vi "LHF.DB.Mongo.Collection.JSON.Aggregate.vi"(6 "Extract _id (T)":bool=TRUE, 8 "error in (no error)":errorcluster, 9 "Operations":variant[](array[variant]), 10 "Collection":string, 11 "LHF.DB.Mongo in":refnum<class "LHF.DB.Mongo.lvclass">) -> (0 "error out":errorcluster, 1 "_id Array":string[](array[string]), 2 "Documents":string[](array[string]), 3 "LHF.DB.Mongo out":refnum<class "LHF.DB.Mongo.lvclass">)   [LabVIEW 2013, in "LHF.DB.Mongo.lvclass"]
doc: "return type: wire cluster of expected document output, then variant to data with documents output. use cluster element's name to choose what document field you're expecting\noperations: wire array of cluster variant, name the cluster variant with the desired aggregation operation as $project or $match then use element names to setup pipeline."
uses:
  LHF.DB.Mongo.lvclass
  C:/Users/Ricardo/Desktop/Projetos/LabVIEW-MongoDB/src/Driver/MongoDB.Bson.dll
  Driver/MongoDB.Bson.dll
  <userlib>/_OpenG.lib/string/string.llb/Trim Whitespace (String)__ogtk.vi
  <vilib>/Utility/VariantDataType/VariantType.lvlib
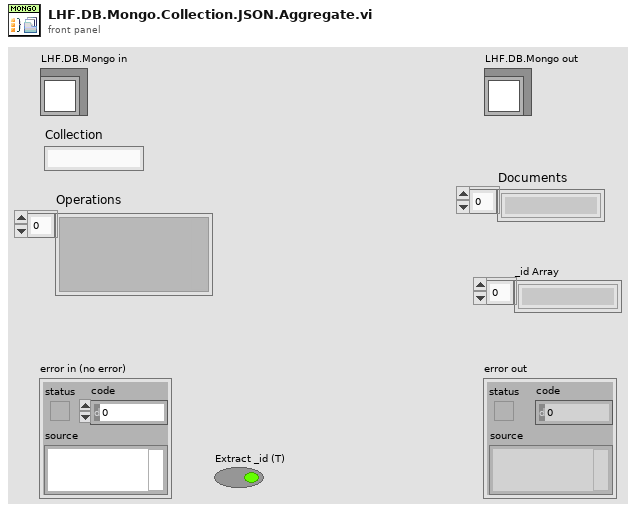
[diagram p1: front panel]
types:
  T1 = enum16{"$project", "$limit", "$skip", "$match", "$redact", "$unwind", "$group", "$sort", "$sample", "$geonear", "$lookup", "$out", "$indexstats"}
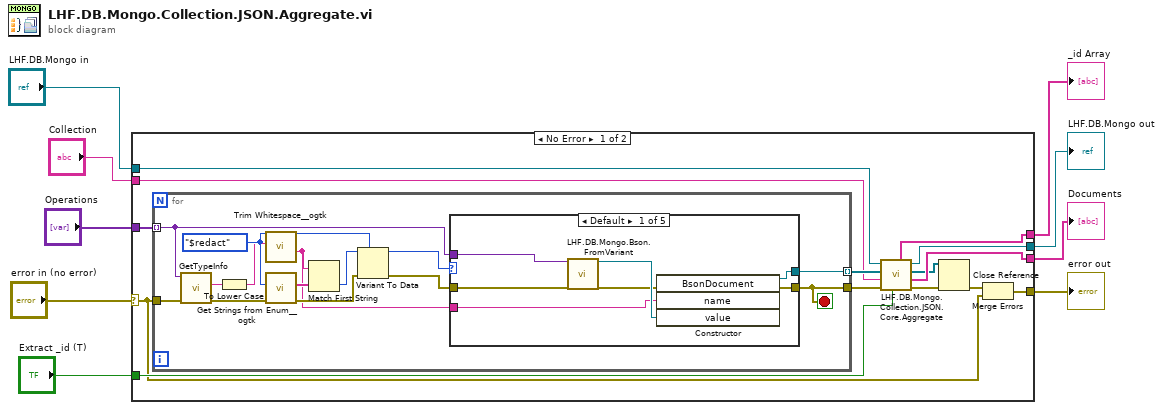
[diagram p0: block diagram]
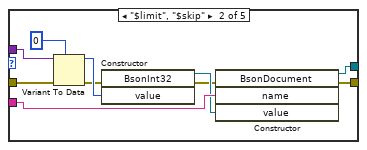
[diagram p2: hidden frame]
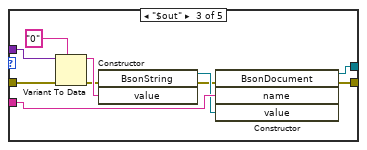
[diagram p3: hidden frame]
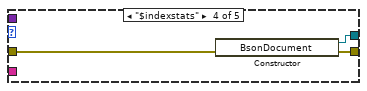
[diagram p4: hidden frame]
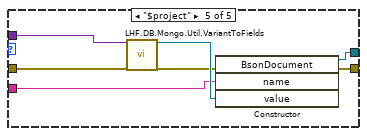
[diagram p5: hidden frame]
diagram:
  n1 = case shown="No Error" "error in (no error)" {
    selector: "error in (no error)" -> [w10 w76]
    tunnel: [w18 w76] -> w8
    tunnel: [w21 w75] -> w6
    tunnel: "LHF.DB.Mongo in" -> [w22 w75]
    tunnel: "Collection" -> [w17 _]
    tunnel: "Operations" -> [w23 _]
    tunnel: [w16 _] -> w3
    tunnel: "Extract _id (T)" -> [w15 _]
    tunnel: [w14 _] -> w1
    frame No Error {
      n2 = for {
        tunnel: w23 -> [w35] mode=indexing
        tunnel: [w37] -> w19 mode=indexing
        tunnel: [w36] -> w20
        tunnel: w10 -> [w29]
        stop <- w36 stop-if-true
        w34 = T1."$redact"
        n3 = call <vilib>:"GetTypeInfo.vi"("error in (no error)"=w29, "Variant"=w35) -> ("error out"=w30:errorcluster, "Name"=w32:string)  [unwired: 5 in, 3 out]
        n4 = To Lower Case(string=w32) -> (all lower case string=w25:string)
        n5 = call-poly <userlib>:"Trim Whitespace__ogtk.vi"("String in"=w25) -> ("String out"=w24:string)  [unwired: 6 in]
        n6 = call <userlib>:"Get Strings from Enum__ogtk.vi"("error in (no error)"=w30, "Enum"=w34) -> ("error out"=w31:errorcluster, "Enum Strings"=w27:string[])  [unwired: 6 in, 2 out]
        n7 = Match First String(2:w27, 3:w24) -> (0:w33:i32)  [unwired: 1 out]
        n8 = Variant To Data(error in=w31, type=w34, Variant=w33) -> (data=w26:T1, error out=w28:errorcluster)
        n9 = case shown="Default" w26 {
          tunnel: [w40 w50 w60 w67 w70] -> w37
          tunnel: [w39 w45 w55 w66 w69] -> w36
          tunnel: w28 -> [w43 w52 w62 w65 w74]
          tunnel: w35 -> [w44 w54 w64 _ w73]
          tunnel: w24 -> [w38 w51 w61 _ w68]
          frame Default {
            n10 = call "LHF.DB.Mongo.Bson.FromVariant.vi"("Variant"=w44, "error IO"=w43) -> ("BsonValue"=w42:refnum<k24>, "error IO 2"=w41:errorcluster)  [unwired: 16 in]
            n11 = constructor class="BsonDocument"(error in=w41, "name"=w38, "value"=w42) -> (reference out=w40:refnum<k24>, error out=w39:errorcluster)  [unwired: 2 in, 3 out]
          }
          frame "$limit", "$skip" {
            n12 = Variant To Data(error in=w52, type=0, Variant=w54) -> (data=w49:i32, error out=w48:errorcluster)
            n13 = constructor class="BsonInt32"(error in=w48, "value"=w49) -> (reference out=w47:refnum<k24>, error out=w46:errorcluster)  [unwired: 2 in, 2 out]
            n14 = constructor class="BsonDocument"(error in=w46, "name"=w51, "value"=w47) -> (reference out=w50:refnum<k24>, error out=w45:errorcluster)  [unwired: 2 in, 3 out]
          }
          frame "$out" {
            n15 = Variant To Data(error in=w62, type="0", Variant=w64) -> (data=w59:string, error out=w58:errorcluster)
            n16 = constructor class="BsonString"(error in=w58, "value"=w59) -> (reference out=w57:refnum<k24>, error out=w56:errorcluster)  [unwired: 2 in, 2 out]
            n17 = constructor class="BsonDocument"(error in=w56, "name"=w61, "value"=w57) -> (reference out=w60:refnum<k24>, error out=w55:errorcluster)  [unwired: 2 in, 3 out]
          }
          frame "$indexstats" {
            n18 = constructor class="BsonDocument"(error in=w65) -> (reference out=w67:refnum<k24>, error out=w66:errorcluster)  [unwired: 2 in, 1 out]
          }
          frame "$project" {
            n19 = call "LHF.DB.Mongo.Util.VariantToFields.vi"("projection type"=w73, "error in (no error)"=w74) -> ("BsonDocument"=w72:refnum<k24>, "error out"=w71:errorcluster)  [unwired: 16 in]
            n20 = constructor class="BsonDocument"(error in=w71, "name"=w68, "value"=w72) -> (reference out=w70:refnum<k24>, error out=w69:errorcluster)  [unwired: 2 in, 3 out]
          }
        }
      }
      n21 = call "LHF.DB.Mongo.Collection.JSON.Core.Aggregate.vi"("Extract _id"=w15, "error in (no error)"=w20, "Collection"=w17, "operations"=w19, "LHF.DB.Mongo in"=w22) -> ("error out"=w12:errorcluster, "JSON Documents"=w16:string[], "operations out"=w13:refnum<k24>[], "LHF.DB.Mongo out"=w21:refnum<class "LHF.DB.Mongo.lvclass">, "_id Array"=w14:string[])  [unwired: 2 in]
      n22 = Close Reference(reference=w13, error in (no error)=w12) -> (error out=w11:errorcluster)
      n23 = Merge Errors(w11, w10) -> (w18:errorcluster)
    }
    frame Error {
    }
  }
  "error out" <- w8
  "LHF.DB.Mongo out" <- w6
  "Documents" <- w3
  "_id Array" <- w1
